vi "convert 1D image array to 2D image - polymorphic.vi"   [LabVIEW 2018]
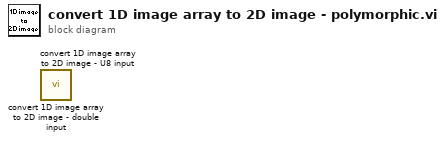
[diagram p0: block diagram]
diagram:
  n1 = call "convert 1D image array to 2D image - double input.vi"() -> ()  [unwired: 11 in, 1 out]
  n2 = call "convert 1D image array to 2D image - U8 input.vi"() -> ()  [unwired: 11 in, 1 out]
